vi "Axes Write.vi"(4 "error in (no error)":errorcluster, 5 "Value":T3, 6 "Container State":T2, 7 "Display State In":T1) -> (0 "error out":errorcluster, 3 "Display State Out":T1)   [LabVIEW 2017, in "XListGraph.lvlib" / "XListGraph.xctl"]
uses:
  XListGraph.xctl
  <vilib>/_xctls/Container State.ctl
  Ability/State.ctl
  Support/def-XListGraphOper.ctl
  <vilib>/_xctls/XControlSupport.lvlib
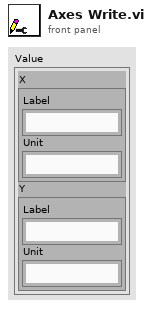
[diagram p1: front panel]
types:
  T1 = typedef "XListGraph.lvlib/XListGraph.xctl/State.ctl" = cluster{"ListWindowSpliterPos":i32, "ListWindowSpliterLocked":bool, "axes":cluster{"X":cluster{"Label":string, "Unit":string}, "Y":cluster{"Label":string, "Unit":string}}, "Next State":string, "User Event":refnum<user-event>, "Plot Names":string[], "Visible Plot Names":string[], "Selected Plot Names":string[]}
  T2 = typedef "XControlSupport.lvlib/Container State.ctl" = cluster{"Indicator?":bool, "Run Mode?":bool, " Refnum":refnum<vi>}
  T3 = cluster{"X":cluster{"Label":string, "Unit":string}, "Y":cluster{"Label":string, "Unit":string}}
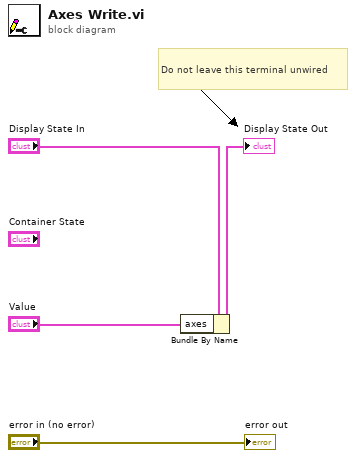
[diagram p0: block diagram]
diagram:
  # "Do not leave this terminal unwired"
  n1 = Bundle By Name(cluster="Display State In", "axes"="Value") -> (→"Display State Out":T1)
  "error out" <- "error in (no error)"
